vi "Fabonacci.vi"() -> ()   [LabVIEW 2020]
panel:
  out "Array":dbl[](array[numeric])
  in  "COUNT":dbl
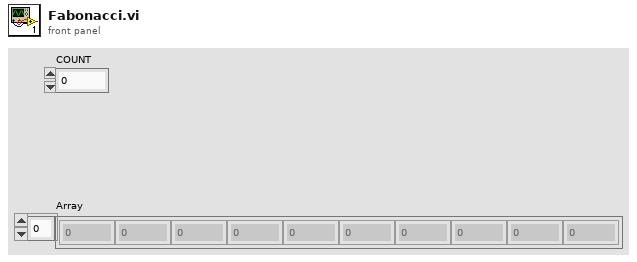
[diagram p1: front panel]
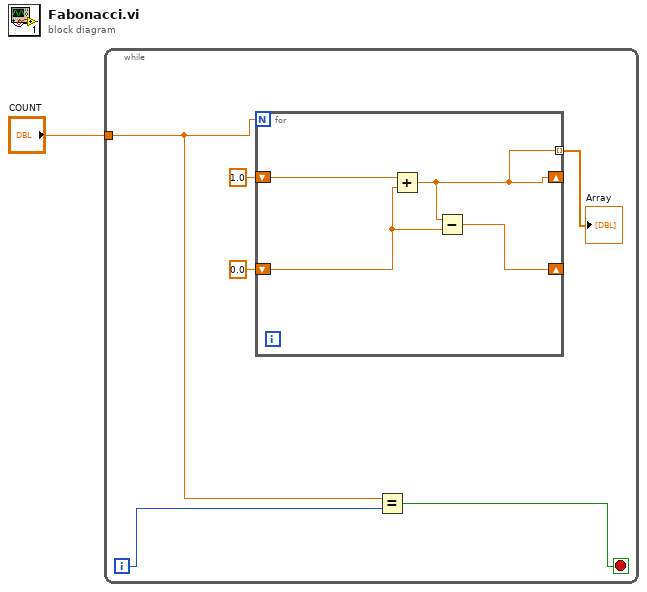
[diagram p0: block diagram]
diagram:
  n1 = while {
    tunnel: "COUNT" -> [w5]
    i -> [w6]
    stop <- w7 stop-if-true
    n2 = for {
      N: w5 -> [_]
      shift-right: [w8] -> _
      shift-left: 1.0 -> [w10]
      shift-right: [w11] -> _
      shift-left: 0.0 -> [w9]
      tunnel: [w8] -> w4 mode=indexing
      n3 = Add(x=w10, y=w9) -> (x+y=w8:dbl)
      n4 = Subtract(x=w8, y=w9) -> (x-y=w11:dbl)
    }
    "Array" <- w4
    n5 = Equal?(x=w5, y=w6) -> (x = y?=w7:bool)
  }
